vi "Bootloader - Close Communication (COM).vi"(0 "COM Port":refnum<visa-resource-name>="COMx", 11 "error in (no error)":errorcluster) -> (15 "error out":errorcluster)   [LabVIEW 2010]
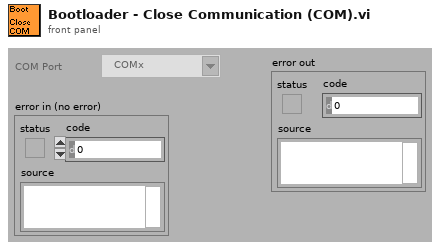
[diagram p1: front panel]
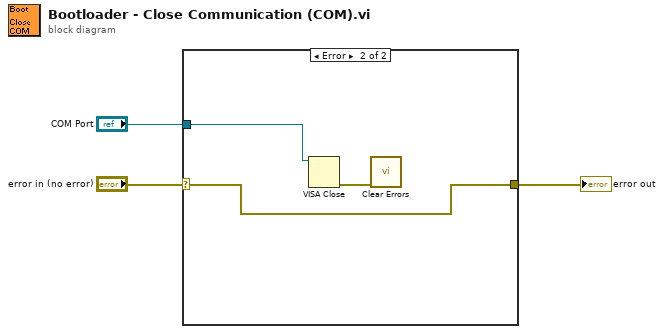
[diagram p0: block diagram]
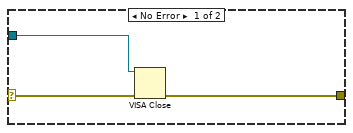
[diagram p2: hidden frame]
diagram:
  n1 = case shown="Error" "error in (no error)" {
    selector: "error in (no error)" -> [w4 w7]
    tunnel: "COM Port" -> [w6 w9]
    tunnel: [w5 w7] -> w2
    frame No Error {
      n2 = VISA Close(VISA resource name=w6, error in (no error)=w4) -> (error out=w5:errorcluster)
    }
    frame Error {
      n3 = VISA Close(VISA resource name=w9) -> (error out=w8:errorcluster)  [unwired: 1 in]
      n4 = call <vilib>:"Clear Errors.vi"("error in (no error)"=w8) -> ()  [unwired: 6 in, 1 out]
    }
  }
  "error out" <- w2
